vi "Configure Trigger (Slope).vi"(0 "VISA resource name":refnum<visa-resource-name>, 2 "Trigger Source (1: Channel 1)":u16(ring)=1 items=["Channel 1"=1, "Channel 2"=2, "Channel 3"=3, "Channel 4"=4, "Ext"=5, "Ext5"=6], 5 "Trigger Level (0.0 V)":dbl, 9 "Holdoff Type (4: IS)":u16(ring)=4 items=["TI", "PS", "PL", "PE", "IS", "IL", "IE"], 11 "error in (no error)":errorcluster, 12 "Slope Time (20 ns)":dbl=2e-08) -> (4 "VISA resource name out":refnum<visa-resource-name>, 15 "error out":errorcluster)   [LabVIEW 2021, in "Siglent SDS 1000 2000 Series.lvlib"]
doc: "Configures slope trigger settings.Slope trigger activates a trigger when the rising or falling edge of a pulse crosses two threshold levels: an upper level and a lower level. The pulse edge must cross the thresholds faster or slower than a selected period of time."
uses:
  <instrlib>/Siglent SDS 1000 2000 Series/Siglent SDS 1000 2000 Series.lvlib
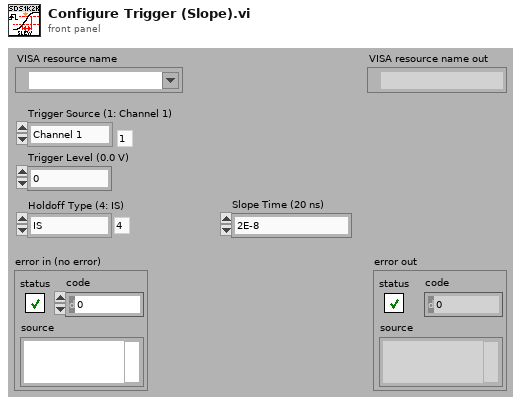
[diagram p1: front panel]
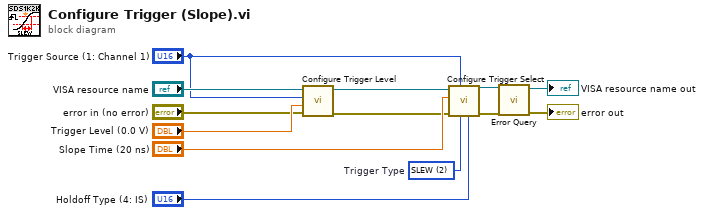
[diagram p0: block diagram]
diagram:
  w5 = u16 2 items=["Edge", "Glitch", "SLEW", "TV"]  # Trigger Type
  n1 = call <instrlib>:"Configure Trigger Level.vi"("error in (no error)"="error in (no error)", "Trigger Level  (0.0 V)"="Trigger Level (0.0 V)", "Channel (1: Channel 1)"="Trigger Source (1: Channel 1)", "VISA resource name"="VISA resource name") -> ("error out"=w1:errorcluster, "VISA resource name out"=w2:refnum<visa-resource-name>)  [unwired: 6 in]
  n2 = call <instrlib>:"Configure Trigger Select.vi"("Hold Type (0: TI)"="Holdoff Type (4: IS)", "Trigger type"=w5, "Trigger Source (1: Channel 1)"="Trigger Source (1: Channel 1)", "error in (no error)"=w1, "Hold Value (100 ns)"="Slope Time (20 ns)", "VISA resource name"=w2) -> ("error out"=w7:errorcluster, "VISA resource name out"=w8:refnum<visa-resource-name>)  [unwired: 4 in]
  n3 = call <instrlib>:"Error Query.vi"("error in (no error)"=w7, "VISA resource name"=w8) -> ("error out"=→"error out":errorcluster, "VISA resource name out"=→"VISA resource name out":refnum<visa-resource-name>)  [unwired: 6 in, 2 out]
